vi "NN_trainer.vi"() -> ()   [LabVIEW 2023]
uses:
  <vilib>/Ngene/Deep Learning Toolkit/Toolkit/NN_Data/API/DataSet_Types/NN_DataSet(In1D_Out1D).ctl
  <vilib>/Ngene/Deep Learning Toolkit/Toolkit/NN_Data/API/DataRef_Types/NN_Data_ref(2D_SGL).ctl
  <vilib>/Ngene/Deep Learning Toolkit/Toolkit/NN_Train/Controls/NN_Train_Session_Data.ctl
  <vilib>/Ngene/Deep Learning Toolkit/Toolkit/NN_Layers/Layers/Input/Controls/NN_Layer_Config(Input1D).ctl
  <vilib>/Ngene/Deep Learning Toolkit/Toolkit/NN_Layers/Layers/FC/Controls/NN_Layer_Config(FC).ctl
  <vilib>/Ngene/Deep Learning Toolkit/Toolkit/NN_Layers/Layers/BatchNorm/Controls/NN_BN_Params.ctl
  <vilib>/Ngene/Deep Learning Toolkit/Toolkit/NN_Activations/Controls/NN_Activation_Type.ctl
  <vilib>/Ngene/Deep Learning Toolkit/Toolkit/NN_Layers/Controls/NN_Layer_Init_Params.ctl
  <vilib>/Ngene/Deep Learning Toolkit/Toolkit/NN_Layers/Controls/NN_Layer_Weight_Init_Type.ctl
  <vilib>/Ngene/Deep Learning Toolkit/Toolkit/NN_Train/Controls/NN_Train_Params.ctl
  <vilib>/Ngene/Deep Learning Toolkit/Toolkit/NN_Train/Controls/NN_Train_Optimizer.ctl
  <vilib>/Ngene/Deep Learning Toolkit/Toolkit/NN_Train/Controls/NN_Train_Data_Sampling.ctl
  <vilib>/Ngene/Deep Learning Toolkit/Toolkit/NN_Train/Controls/NN_LR_Policy_Cfg.ctl
  <vilib>/Ngene/Deep Learning Toolkit/Toolkit/NN_Train/Controls/NN_LR_Policy_Type.ctl
  <vilib>/Ngene/Deep Learning Toolkit/Toolkit/NN_Layers/Layers/Input/NN_Layer_Create(Input1D).vi
  <vilib>/Ngene/Deep Learning Toolkit/Toolkit/NN_Layers/Layers/FC/NN_Layer_Create(FC).vi
  <vilib>/Ngene/Deep Learning Toolkit/Toolkit/NN_Train/Loss_Functions/NN_Set_Loss(MSE).vi
  <vilib>/Utility/file.llb/Read Delimited Spreadsheet (DBL).vi
  <vilib>/Ngene/Deep Learning Toolkit/Toolkit/NN_Train/SubVIs/Dataset_Checks/NN_Check_Dataset(In1D_Out1D).vi
  <vilib>/Ngene/Deep Learning Toolkit/Toolkit/NN_Data/subVIs/Dataset_Split/NN_DataSet_Split(In1D_Out1D).vi
  <vilib>/Ngene/Deep Learning Toolkit/Toolkit/NN_Network/subVIs/NN_Predict/NN_Predict(In1D_Out1D).vi
  <vilib>/Ngene/Deep Learning Toolkit/Toolkit/NN_Train/Eval_Loss/NN_Eval_Test_Error_Loss/NN_Eval(In1D_Out1D).vi
  <vilib>/Ngene/Deep Learning Toolkit/Toolkit/Deep_Learning_Toolkit_by_Ngene.lvlib
panel:
  out "Loss":sgl(graph)
  out "Predictions":sgl[][](array[numeric])
  in  "stop":bool
  out "Session Data":T1
  out "Labels":sgl[][](array[numeric])
  out "Features":sgl[][](array[numeric])
  out "Epoch_num":i32
  out "Eval Losses":sgl[](array[numeric])
  out "Epoch Test Loss":sgl
  out "Epoch Train Loss":sgl
  out "Eval Size":i32
  out "Train Size":i32
  out "Dataset Train":T2
  out "Dataset Eval":T2
  out "all rows":dbl[][](array[numeric])
  out "Iter":i32=57524
  in  "file path (dialog if empty)":path=path "C:/Users/sebas/OneDrive/Documents/EPFLRT/TorqueAllocationNN/data/TA_data.csv"
  out "error out 2":errorcluster
  out "error out":errorcluster
  out "Train Lossese":sgl[](array[numeric])
  in  "Working Dir":path=path "C:/Users/sebas/OneDrive/Documents/EPFLRT/TorqueAllocationNN/models/LabVIEW"
  out "CFG File Path":path
  out "Weight Path out":path
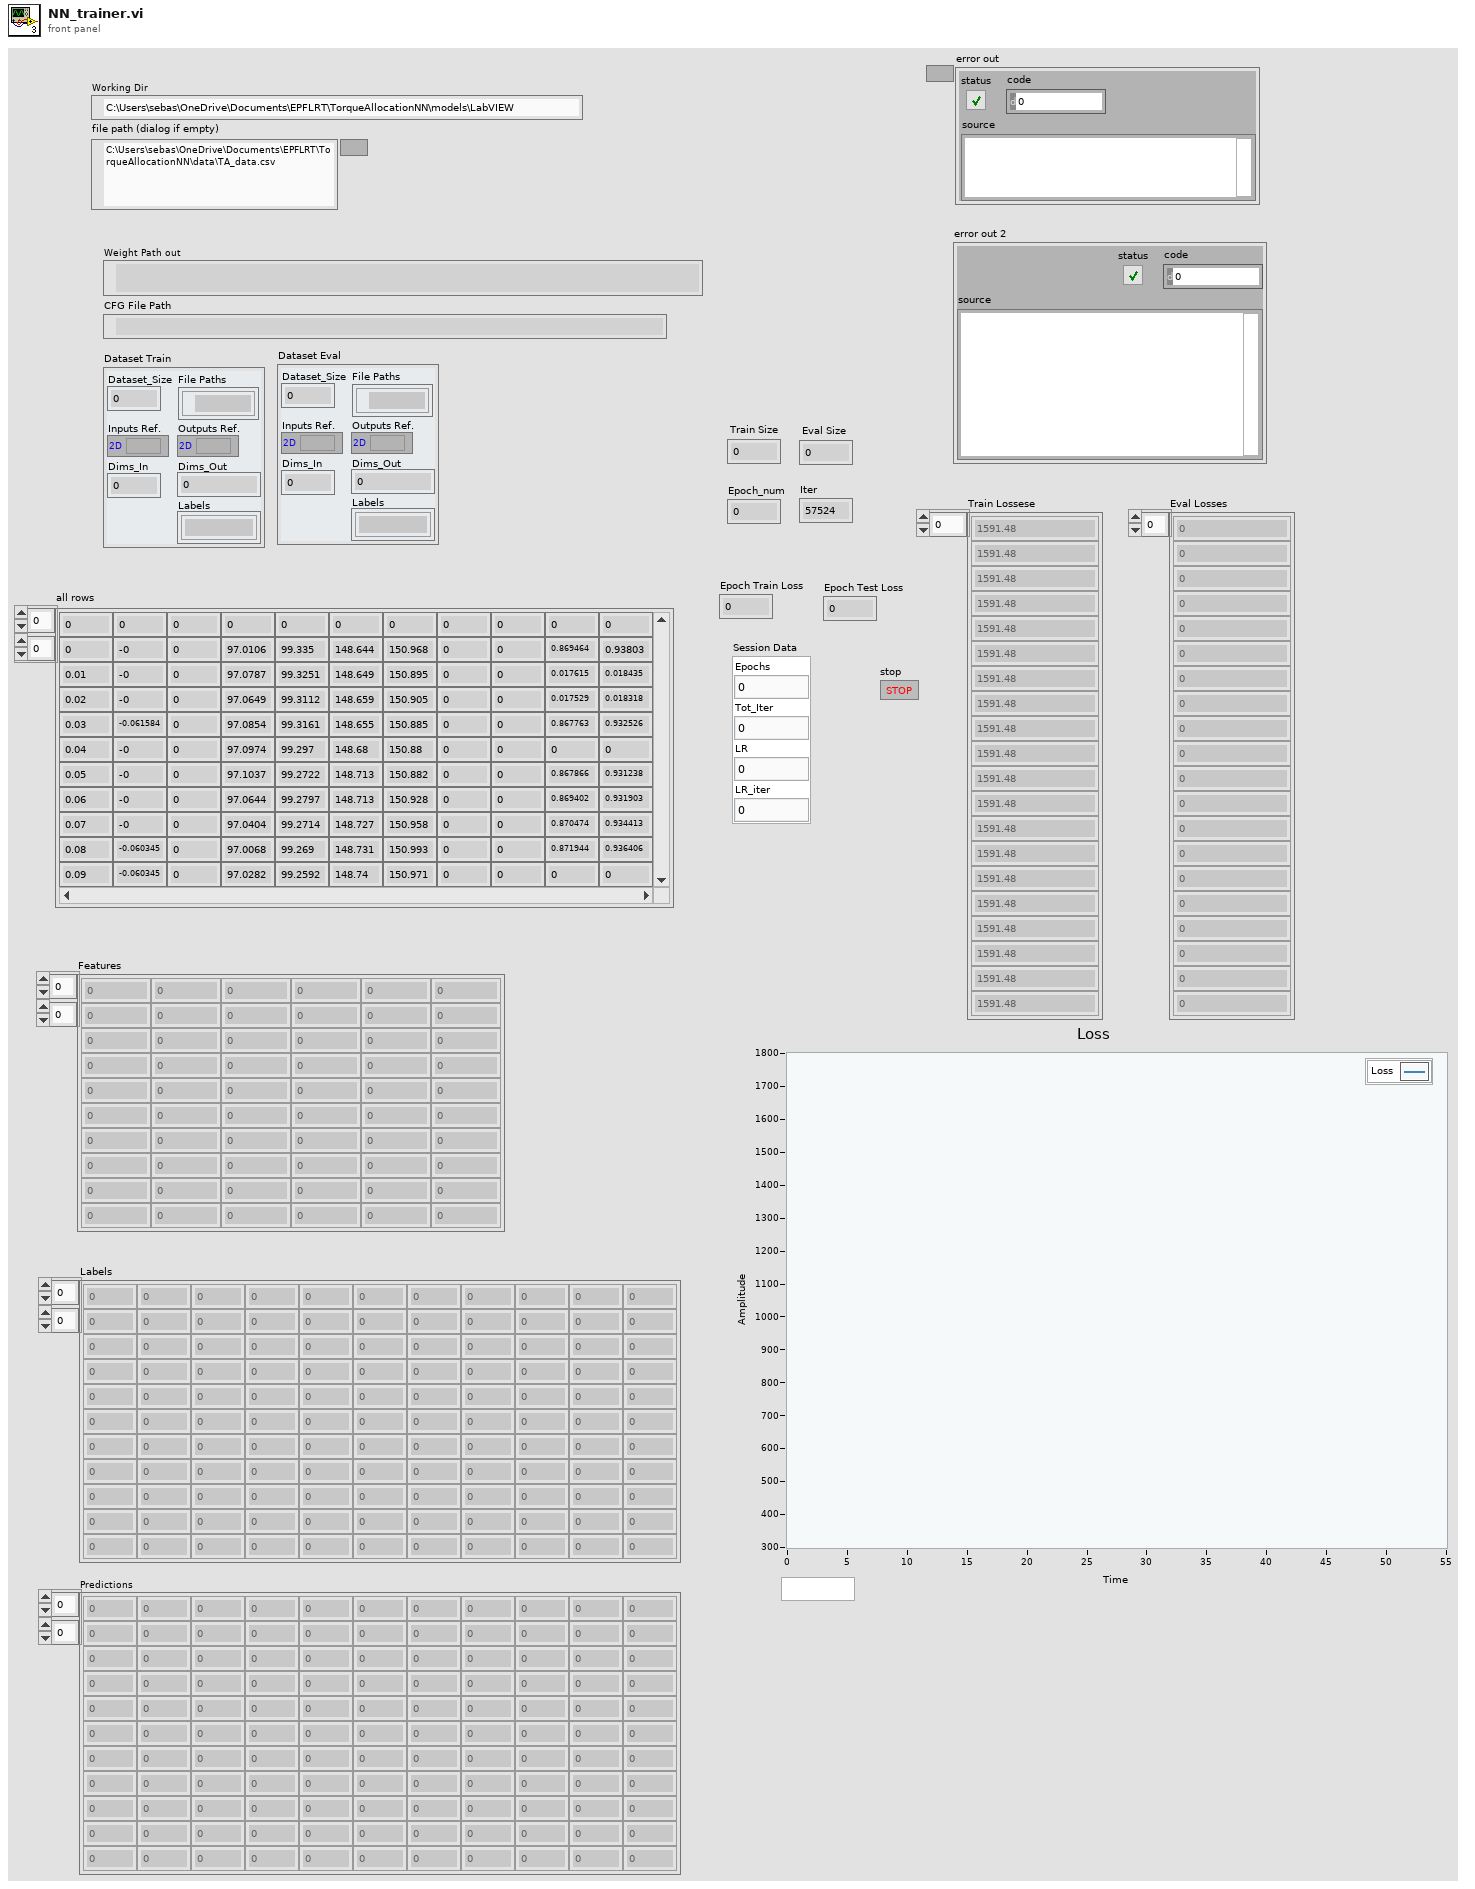
[diagram p1: front panel]
types:
  T1 = typedef "Deep_Learning_Toolkit_by_Ngene.lvlib/NN_Train_Session_Data.ctl" = cluster{"Epochs":sgl, "Tot_Iter":i32, "LR":sgl, "LR_iter":i32}
  T2 = typedef "Deep_Learning_Toolkit_by_Ngene.lvlib/NN_DataSet(In1D_Out1D).ctl" = cluster{"Inputs Ref.":T3, "Outputs Ref.":T3, "Dims_In":i32, "Dataset_Size":i32, "Dims_Out":i32, "Labels":string[], "File Paths":path[]}
  T3 = typedef "Deep_Learning_Toolkit_by_Ngene.lvlib/NN_Data_ref(2D_SGL).ctl" = refnum<data-value>
  T4 = typedef "Deep_Learning_Toolkit_by_Ngene.lvlib/NN_LR_Policy_Cfg.ctl" = cluster{"Policy_Type":T5, "LR0":dbl, "k":sgl, "WarmUp_Policy":enum16{"Step", "Ramp"}, "WarmUp_Iter":i32, "WarmUp_Ratio":sgl}
  T5 = typedef "Deep_Learning_Toolkit_by_Ngene.lvlib/NN_LR_Policy_Type.ctl" = enum16{"Manual", "Step", "Exp", "1/t"}
  T6 = typedef "Deep_Learning_Toolkit_by_Ngene.lvlib/NN_Train_Params.ctl" = cluster{"Optimizer":T7, "Beta_1":sgl, "Beta_2":sgl, "Weight Decay(L1)":sgl, "Weight Decay(L2)":sgl, "Data_Sampling":T8}
  T7 = typedef "Deep_Learning_Toolkit_by_Ngene.lvlib/NN_Train_Optimizer.ctl" = enum16{"SGD", "Adam", "Adagrad", "Adadelta", "RMSProp", "Nesterov"}
  T8 = typedef "Deep_Learning_Toolkit_by_Ngene.lvlib/NN_Train_Data_Sampling.ctl" = enum16{"Random", "Sequential"}
  T9 = typedef "Deep_Learning_Toolkit_by_Ngene.lvlib/NN_Layer_Config(FC).ctl" = cluster{"Name":string, "Size":i32, "BN":bool, "BN_Params":T10, "Activation":T11, "Has Bias?":bool, "Init_Params":T12, "Custom_Params":string}
  T10 = typedef "Deep_Learning_Toolkit_by_Ngene.lvlib/NN_BN_Params.ctl" = cluster{"epsilon":sgl, "momentum":sgl}
  T11 = typedef "Deep_Learning_Toolkit_by_Ngene.lvlib/NN_Activation_Type.ctl" = enum16{"Sigmoid", "ReLU", "LReLU", "ReLU6", "tanh", "Swish", "Mish", "None"}
  T12 = typedef "Deep_Learning_Toolkit_by_Ngene.lvlib/NN_Layer_Init_Params.ctl" = cluster{"Init_Type":T13, "Value":sgl}
  T13 = typedef "Deep_Learning_Toolkit_by_Ngene.lvlib/NN_Layer_Weight_Init_Type.ctl" = enum16{"Const", "Uniform", "Gaussian", "Xavier"}
  T14 = typedef "Deep_Learning_Toolkit_by_Ngene.lvlib/NN_Layer_Config(Input1D).ctl" = cluster{"Name":string, "Size":i32}
  T15 = typedef "Deep_Learning_Toolkit_by_Ngene.lvlib/NN.ctl" = cluster{"Name":string, "No of Layers":i32, "mBatch":i32, "Layers":T16[], "Dimty":T17, "Dims_In":T18, "Dims_Out":T18, "Working_Dir":path, "Train?":bool, "Train_Params":T6, "LR_Update_Policy":T4, "Session Data":T1, "Ground_truth":T19, "NNg_hdls":T20, "NN_Device":T21, "GPU Id":i32, "Labels":string[], "Receptive Field":T22[], "Loss_Type":T23, "Loss_Cfg_Prms":variant, "NNG_WS":T24}
  T16 = typedef "Deep_Learning_Toolkit_by_Ngene.lvlib/NN_Layer_ref.ctl" = refnum<data-value>
  T17 = typedef "Deep_Learning_Toolkit_by_Ngene.lvlib/NN_In_Out_Dim-ty.ctl" = enum8{"In1D_Out1D", "In3D_Out1D", "In3D_Out3D", "In3D_OutBBox"}
  T18 = typedef "Deep_Learning_Toolkit_by_Ngene.lvlib/NN_Dims(C,H,W).ctl" = cluster{"C":i32, "H":i32, "W":i32}
  T19 = typedef "Deep_Learning_Toolkit_by_Ngene.lvlib/NN_Ground_truth.ctl" = cluster{"Y":variant}
  T20 = typedef "Deep_Learning_Toolkit_by_Ngene.lvlib/nng_cuda_handles.ctl" = cluster{"cudnn":u64, "cublas":u64, "stream":u64, "curand":u64}
  T21 = typedef "Deep_Learning_Toolkit_by_Ngene.lvlib/NN_Device.ctl" = enum16{"CPU", "GPU"}
  T22 = typedef "Deep_Learning_Toolkit_by_Ngene.lvlib/NN_Dims(V,H).ctl" = cluster{"V":i32, "H":i32}
  T23 = typedef "Deep_Learning_Toolkit_by_Ngene.lvlib/NN_Loss_Type.ctl" = enum16{"None", "MSE", "CrossEntropy", "YOLO_v2", "YOLO_v4"}
  T24 = typedef "Deep_Learning_Toolkit_by_Ngene.lvlib/NNG_WS.ctl" = cluster{"NNG_WS_Mem":T25, "Max_WS_Size":i64}
  T25 = typedef "Deep_Learning_Toolkit_by_Ngene.lvlib/NNg_WS_Mem_DVR.ctl" = refnum<data-value>
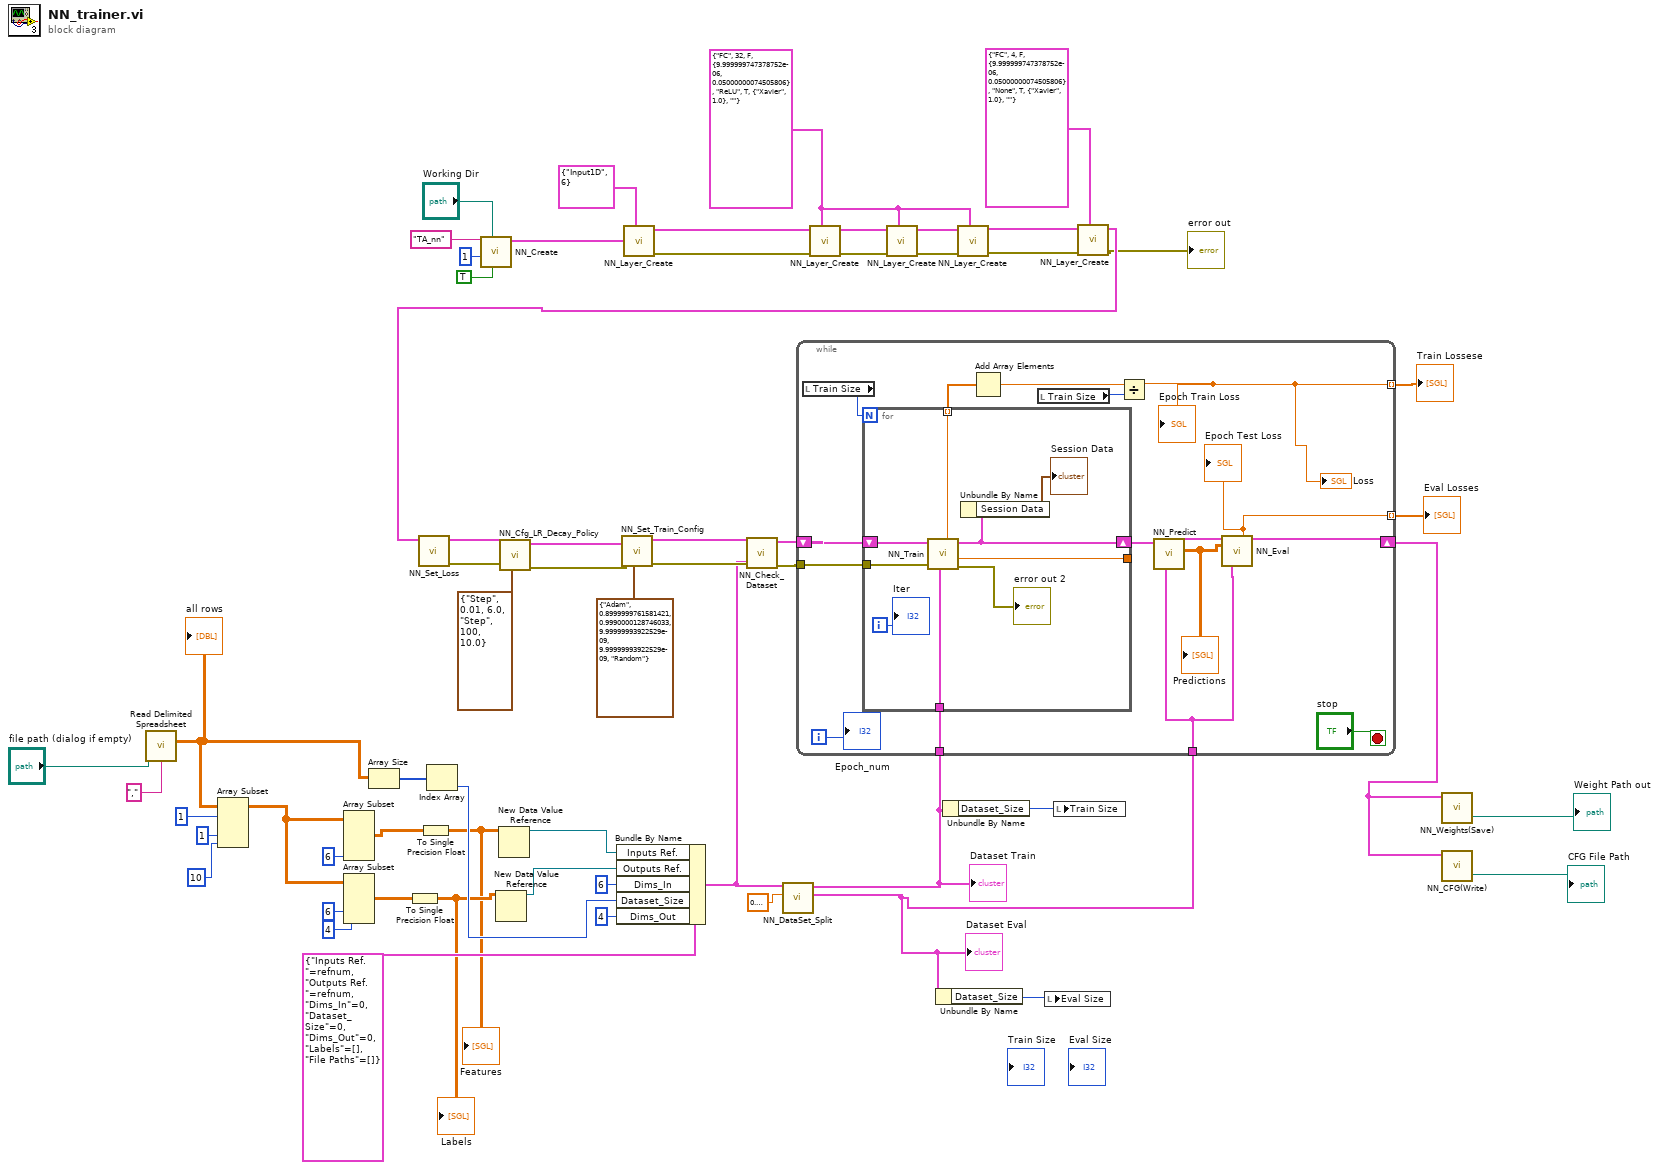
[diagram p0: block diagram]
diagram:
  w47 = T9 {"Name"="FC", "Size"=32, "BN"=FALSE, "BN_Params"={"epsilon"=1e-05, "momentum"=0.05}, "Activation"=enum."ReLU", "Has Bias?"=TRUE, "Init_Params"={"Init_Type"=enum."Xavier", "Value"=1.0}, "Custom_Params"=""} ("FC_Cfg")
  n1 = call-poly <vilib>:"Read Delimited Spreadsheet.vi"("file path (dialog if empty)"="file path (dialog if empty)", "delimiter (\\t)"="," ("delimiter (\\t)")) -> ("all rows"=w22:dbl[][])  [unwired: 8 in, 5 out]
  "all rows" <- w22
  n2 = Array Subset(array=w22, index (row)=1 ("index"), index (col)=1 ("index"), length (col)=10 ("length")) -> (w5:dbl[][])  [unwired: 1 in]
  n3 = Array Subset(array=w5, length (col)=6 ("length")) -> (w19:dbl[][])  [unwired: 3 in]
  n4 = Array Subset(array=w5, index (col)=6 ("index"), length (col)=4 ("length")) -> (w20:dbl[][])  [unwired: 2 in]
  n5 = Array Size(array=w22) -> (size(s)=w29:i32[])
  n6 = To Single Precision Float(number=w20) -> (single precision float=w16:sgl[][])
  "Labels" <- w16
  n7 = To Single Precision Float(number=w19) -> (single precision float=w15:sgl[][])
  "Features" <- w15
  n8 = Index Array(array=w29) -> (element=w28:i32)  [unwired: 1 in]
  n9 = call <vilib>:"NN_Create.vi"("Train? (false)"=TRUE, "Working Dir"="Working Dir", "mBatch (1)"=1, "Name"="TA_nn") -> ("NN out"=w60:T15)  [unwired: 6 in, 1 out]
  n10 = New Data Value Reference(data value=w16) -> (data value reference=w17:refnum<data-value>)  [unwired: 1 in, 1 out]
  n11 = New Data Value Reference(data value=w15) -> (data value reference=w18:refnum<data-value>)  [unwired: 1 in, 1 out]
  n12 = Bundle By Name(cluster=T2 {"Inputs Ref."=refnum, "Outputs Ref."=refnum, "Dims_In"=0, "Dataset_Size"=0, "Dims_Out"=0, "Labels"=[], "File Paths"=[]} ("Dataset(In1D_Out1D)"), "Inputs Ref."=w18, "Outputs Ref."=w17, "Dims_In"=6, "Dataset_Size"=w28, "Dims_Out"=4) -> (w14:T2)
  n13 = call-poly <vilib>:"NN_Layer_Create.vi"("Input1D_Cfg"=T14 {"Name"="Input1D", "Size"=6}, "NN in"=w60) -> ("error out"=w56:errorcluster, "NN out"=w59:T15)  [unwired: 7 in, 1 out]
  n14 = call-poly <vilib>:"NN_DataSet_Split.vi"("Split Size"=sgl 0.2, "Dataset In"=w14) -> ("Dataset Out 2"=w7:T2, "Dataset Out 1"=w10:T2)  [unwired: 7 in, 1 out]
  "Dataset Eval" <- w7
  "Dataset Train" <- w10
  n15 = call-poly <vilib>:"NN_Layer_Create.vi"("FC_Cfg"=w47, "error in (no error)"=w56, "NN in"=w59) -> ("error out"=w55:errorcluster, "NN out"=w58:T15)  [unwired: 6 in, 1 out]
  n16 = call-poly <vilib>:"NN_Layer_Create.vi"("FC_Cfg"=w47, "error in (no error)"=w55, "NN in"=w58) -> ("error out"=w54:errorcluster, "NN out"=w57:T15)  [unwired: 6 in, 1 out]
  n17 = Unbundle By Name(w7) -> ("Dataset_Size"=w6:i32)
  n18 = Unbundle By Name(w10) -> ("Dataset_Size"=w9:i32)
  n19 = call-poly <vilib>:"NN_Layer_Create.vi"("FC_Cfg"=w47, "error in (no error)"=w54, "NN in"=w57) -> ("error out"=w50:errorcluster, "NN out"=w51:T15)  [unwired: 6 in, 1 out]
  n20 = local write "Eval Size"(w6) -> ()
  n21 = local write "Train Size"(w9) -> ()
  n22 = call-poly <vilib>:"NN_Layer_Create.vi"("FC_Cfg"=T9 {"Name"="FC", "Size"=4, "BN"=FALSE, "BN_Params"={"epsilon"=1e-05, "momentum"=0.05}, "Activation"=enum."None", "Has Bias?"=TRUE, "Init_Params"={"Init_Type"=enum."Xavier", "Value"=1.0}, "Custom_Params"=""}, "error in (no error)"=w50, "NN in"=w51) -> ("error out"=→"error out":errorcluster, "NN out"=w43:T15)  [unwired: 6 in, 1 out]
  n23 = call-poly <vilib>:"NN_Set_Loss.vi"("NN in"=w43) -> ("error out"=w35:errorcluster, "NN out"=w42:T15)  [unwired: 9 in]
  n24 = call <vilib>:"NN_Cfg_LR_Decay_Policy.vi"("LR_Decay_Params"=T4 {"Policy_Type"=enum."Step", "LR0"=0.01, "k"=6.0, "WarmUp_Policy"=enum."Step", "WarmUp_Iter"=100, "WarmUp_Ratio"=10.0}, "error in (no error)"=w35, "NN in"=w42) -> ("error out"=w34:errorcluster, "NN out"=w40:T15)  [unwired: 7 in]
  n25 = call <vilib>:"NN_Set_Train_Config.vi"("NN_Train_Params"=T6 {"Optimizer"=enum."Adam", "Beta_1"=0.9, "Beta_2"=0.999, "Weight Decay(L1)"=1e-08, "Weight Decay(L2)"=1e-08, "Data_Sampling"=enum."Random"}, "error in (no error)"=w34, "NN in"=w40) -> ("error out"=w33:errorcluster, "NN out"=w39:T15)  [unwired: 7 in]
  n26 = call-poly <vilib>:"NN_Check_Dataset.vi"("Dataset"=w14, "error in (no error)"=w33, "NN in"=w39) -> ("error out"=w24:errorcluster, "NN out"=w38:T15)  [unwired: 7 in]
  n27 = while {
    tunnel: w24 -> [w75]
    tunnel: [w61] -> w11 mode=indexing
    tunnel: w10 -> [w73]
    shift-right: [w68] -> w37
    shift-left: w38 -> [w76]
    tunnel: w7 -> [w65]
    tunnel: [w62] -> w8 mode=indexing
    i -> [w64]
    stop <- "stop" stop-if-true
    n28 = local read "Train Size"() -> (w71:i32)
    n29 = for {
      N: w71 -> [_]
      tunnel: w73 -> [w83]
      tunnel: w75 -> [w82]
      shift-right: [w79] -> w69
      shift-left: w76 -> [w85]
      tunnel: [w80] -> _
      tunnel: [w77] -> w74 mode=indexing
      i -> [w81]
      n30 = call <vilib>:"NN_Train.vi"("Train Dataset"=w83, "error in (no error)"=w82, "NN in"=w85) -> ("error out"=→"error out 2":errorcluster, "Total"=w80:dbl, "NN out"=w79:T15, "Loss"=w77:sgl)  [unwired: 4 in, 1 out]
      n31 = Unbundle By Name(w79) -> ("Session Data"=→"Session Data":T1)
      "Iter" <- w81
    }
    n32 = Add Array Elements(numeric array=w74) -> (sum=w72:sgl)
    n33 = local read "Train Size"() -> (w70:i32)
    n34 = Divide(x=w72, y=w70) -> (x/y=w61:sgl)
    "Epoch Train Loss" <- w61
    "Loss" <- w61
    n35 = call-poly <vilib>:"NN_Predict.vi"("Dataset"=w65, "NN in"=w69) -> ("Predictions"=w66:sgl[][], "NN out"=w67:T15)  [unwired: 7 in, 1 out]
    "Predictions" <- w66
    n36 = call-poly <vilib>:"NN_Eval.vi"("NN in"=w67, "Predictions"=w66, "Dataset"=w65) -> ("Loss"=w62:sgl, "NN out"=w68:T15)  [unwired: 8 in, 3 out]
    "Epoch Test Loss" <- w62
    "Epoch_num" <- w64
  }
  "Train Lossese" <- w11
  "Eval Losses" <- w8
  n37 = call <vilib>:"NN_Weights(Save).vi"("NN in"=w37) -> ("Weight Path out"=→"Weight Path out":path)  [unwired: 8 in, 2 out]
  n38 = call <vilib>:"NN_CFG(Write).vi"("NN in"=w37) -> ("CFG File Path"=→"CFG File Path":path)  [unwired: 8 in, 2 out]
